vi "Wait Time(with error).vi"(8 "error in":errorcluster, 11 "Wait Time（ms）":u32) -> (0 "error out":errorcluster)   [LabVIEW 2019]
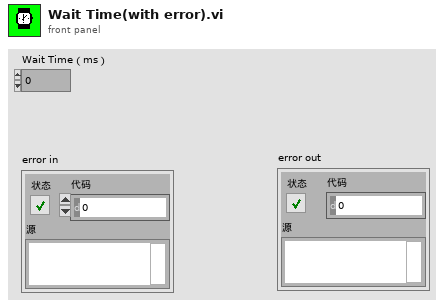
[diagram p1: front panel]
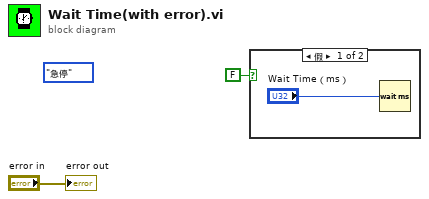
[diagram p0: block diagram]
diagram:
  (unwired) enum16{"停止", "运行", "复位", "急停"}."急停" ("x")
  n1 = case shown="假" FALSE {
    frame False {
      n2 = Wait (ms)(milliseconds to wait="Wait Time（ms）") -> ()  [unwired: 1 out]
    }
    frame True {
    }
  }
  "error out" <- "error in"
